vi "PythonName.vi"(6 "add self":bool=TRUE, 8 "error in":errorcluster, 11 "Diagram in":refnum<class "Diagram.lvclass">) -> (0 "error out":errorcluster, 3 "Diagram out":refnum<class "Diagram.lvclass">, 5 "name":string, 7 "UID":string)   [LabVIEW 2014, in "Diagram.lvclass"]
uses:
  Diagram.lvclass
  Python/Parsing/Python Functions.lvlib
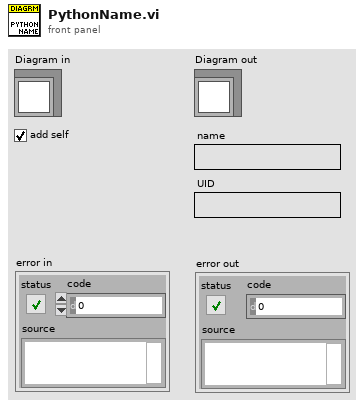
[diagram p1: front panel]
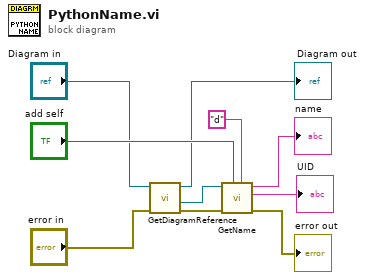
[diagram p0: block diagram]
diagram:
  n1 = call "GetDiagramReference.vi"("error in"="error in", "Diagram in"="Diagram in") -> ("error out"=w5:errorcluster, "reference out"=w4:refnum<vi>, "Diagram out"=→"Diagram out":refnum<class "Diagram.lvclass">)  [unwired: 5 in]
  n2 = call "GetName.vi"("base name"="d", "add self"="add self", "error in"=w5, "GObj Refnum"=w4) -> ("error out"=→"error out":errorcluster, "UID"=→"UID":string, "name"=→"name":string)  [unwired: 5 in]
